vi "Write Cache Manager.vi"(10 "Cache Manager DVR.lvclass":refnum<class "Cache Manager.lvclass">, 11 "Message Flattener in":refnum<class "Message Flattener.lvclass">) -> (3 "Message Flattener out":refnum<class "Message Flattener.lvclass">)   [LabVIEW 2020, in "Message Flattener.lvclass"]
uses:
  Message Flattener.lvclass
  Cache Manager/Cache Manager.lvclass
  Message Flattener.lvclass/Message Flattener.ctl
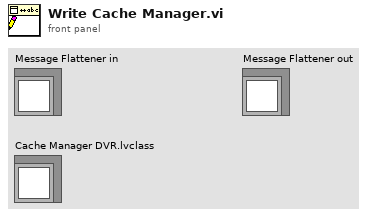
[diagram p1: front panel]
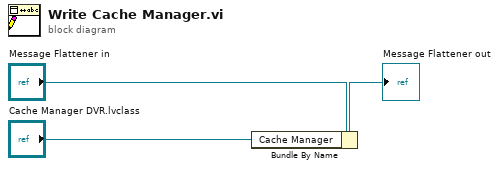
[diagram p0: block diagram]
diagram:
  n1 = Bundle By Name(cluster="Message Flattener in", "Cache Manager"="Cache Manager DVR.lvclass") -> (→"Message Flattener out":refnum<class "Message Flattener.lvclass">)
